vi "NN_Get_Incorrect_Classified_Imgs(RGB)_3D.vi"(4 "# of columns":i32=16, 6 "Dataset":T2={"Inputs Ref."=variant(refnum<data-value> refnum), "Outputs Ref."=refnum, "Dataset_Size"=0, "Dims_In"={"C"=0, "H"=0, "W"=0}, "Dims_Out"=0, "Labels"=[], "File Paths"=[]}, 7 "Labels":string[](array[string]), 8 "error in (no error)":errorcluster, 10 "Predictions":sgl[][](array[numeric]), 11 "MisClassed_idx":i32[](array[numeric])) -> (0 "error out":errorcluster, 3 "Images(GrayScale)":T1[][](array[typedef]))   [LabVIEW 2020]
doc: "Helper VI for analysis.\nReturns Images as intensity graphs with the ground truth and corresponding predictions."
uses:
  <vilib>/Ngene/Deep Learning Toolkit/Toolkit/NN_Data/API/DataSet/DataSet_Types/NN_DataSet(In3D_Out1D).ctl
  <vilib>/Ngene/Deep Learning Toolkit/Toolkit/NN_Data/Controls/DataRef_Types/2D/NN_Data_ref(2D_SGL).ctl
  <vilib>/Ngene/Deep Learning Toolkit/Toolkit/NN_Data/API/NN_Dims(C,H,W).ctl
  Controls/Img_RGB.ctl
  <vilib>/Ngene/Deep Learning Toolkit/Toolkit/NN_Data/subVIs/Dataset/NN_Variant_to_DVR/4D/NN_Data_Variant_to_DVR(4D_SGL).vi
  <vilib>/picture/picture.llb/Draw True-Color Pixmap.vi
  <vilib>/Ngene/Deep Learning Toolkit/Toolkit/Deep_Learning_Toolkit_by_Ngene.lvlib
  <vilib>/vision/NI_Vision_Development_Module.lvlib
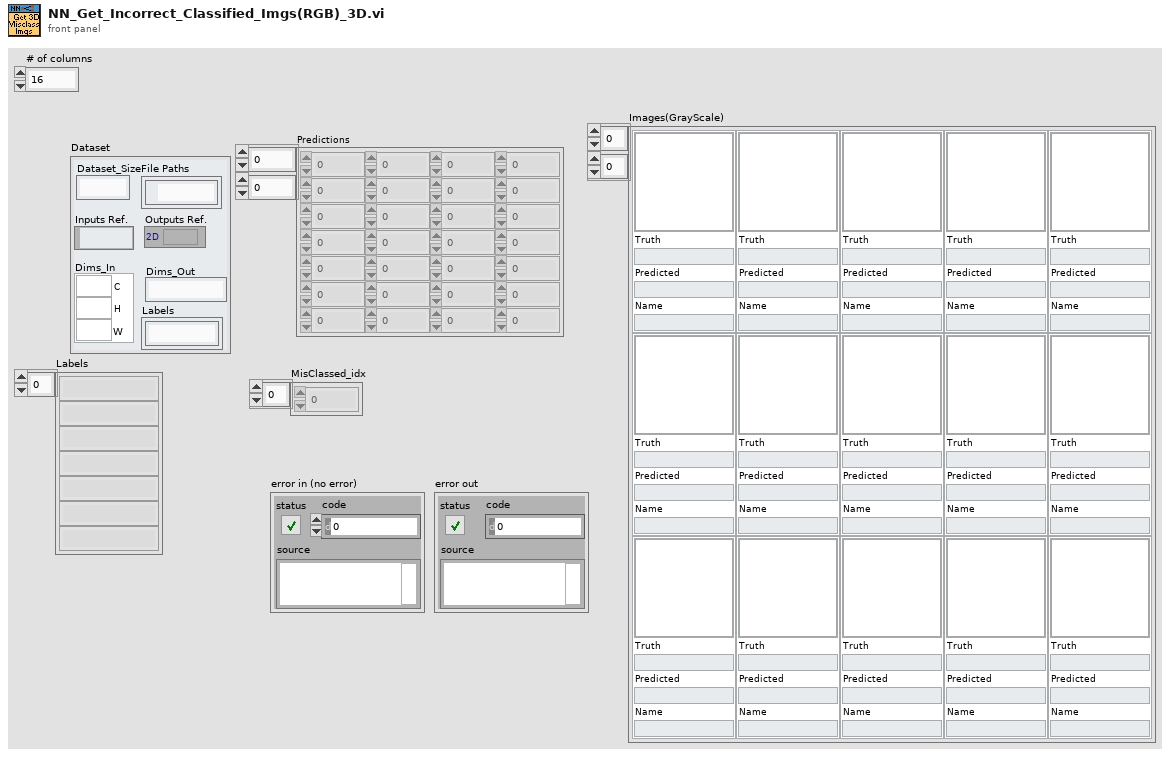
[diagram p1: front panel]
types:
  T1 = typedef "Img_RGB.ctl" = cluster{"image":picture, "Truth":string, "Predicted":string, "Name":string}
  T2 = typedef "Deep_Learning_Toolkit_by_Ngene.lvlib/NN_DataSet(In3D_Out1D).ctl" = cluster{"Inputs Ref.":variant, "Outputs Ref.":T3, "Dataset_Size":i32, "Dims_In":T4, "Dims_Out":i32, "Labels":string[], "File Paths":path[]}
  T3 = typedef "Deep_Learning_Toolkit_by_Ngene.lvlib/NN_Data_ref(2D_SGL).ctl" = refnum<data-value>
  T4 = typedef "Deep_Learning_Toolkit_by_Ngene.lvlib/NN_Dims(C,H,W).ctl" = cluster{"C":i32, "H":i32, "W":i32}
  T5 = typedef "Image Type" = u32
  T6 = typedef "Deep_Learning_Toolkit_by_Ngene.lvlib/NN_Data_ref(4D_SGL).ctl" = refnum<data-value>
  T7 = typedef "IMAQ Image.ctl" = refnum<image>
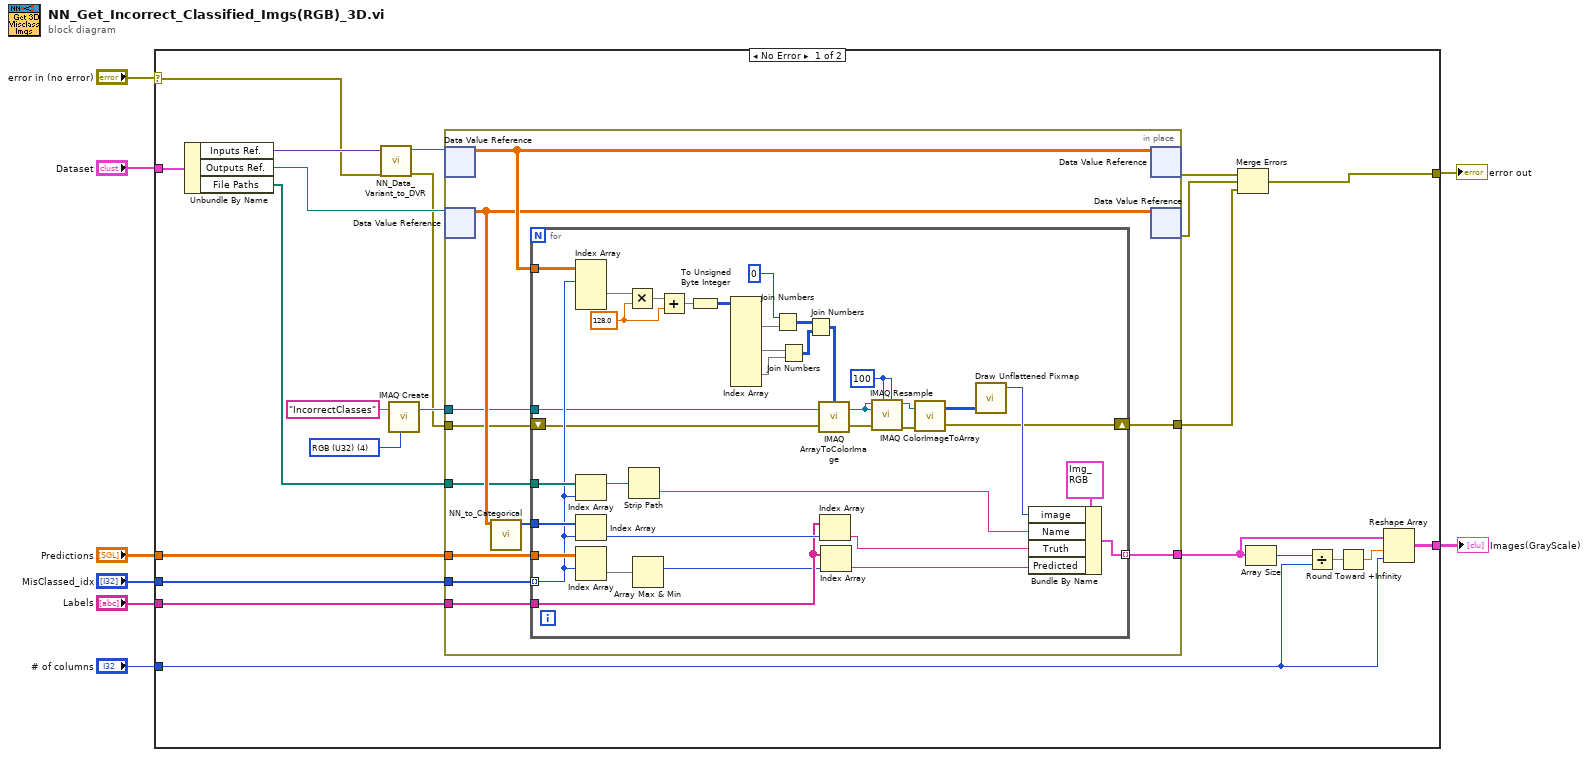
[diagram p0: block diagram]
diagram:
  n1 = case shown="No Error" "error in (no error)" {
    selector: "error in (no error)" -> [w20 w80]
    tunnel: [w31 w80] -> w8
    tunnel: "Dataset" -> [w26 _]
    tunnel: "Predictions" -> [w25 _]
    tunnel: "MisClassed_idx" -> [w24 _]
    tunnel: [w23 _] -> w3
    tunnel: "Labels" -> [w17 _]
    tunnel: "# of columns" -> [w15 _]
    frame No Error {
      w14 = T5 4 items=["Grayscale (U8)", "Grayscale (I16)", "Grayscale (SGL)", "Complex (CSG)", "RGB (U32)", "HSL (U32)", "RGB (U64)", "Grayscale (U16)"] ("Image Type")
      n2 = Unbundle By Name(w26) -> ("Inputs Ref."=w21:variant, "Outputs Ref."=w22:T3, "File Paths"=w16:path[])
      n3 = call-poly <vilib>:"NN_Data_Variant_to_DVR.vi"("error in (no error)"=w20, "Inputs Ref."=w21) -> ("error out"=w11:errorcluster, "DVR(4D_SGL)"=w19:T6)  [unwired: 8 in]
      n4 = call "IMAQ Create"("Image Name"="IncorrectClasses", "Image Type"=w14) -> ("New Image"=w12:T7)  [unwired: 3 in, 1 out]
      n5 = in-place {
        in-place-border: w24 -> [w42]
        in-place-border: w25 -> [w38]
        in-place-border: [w40] -> w27
        in-place-border: w17 -> [w36]
        in-place-border: w16 -> [w35]
        in-place-border: w12 -> [w34]
        in-place-border: w11 -> [w33]
        in-place-border: [w32] -> w10
        n6 = in-place-dvr #1(w19) -> (w41:sgl[][][][])  [unwired: 1 out]
        n7 = in-place-dvr #2(w22) -> (w37:sgl[][])  [unwired: 1 out]
        n8 = call <vilib>:"NN_to_Categorical.vi"("Prediction"=w37) -> ("Label_Idx"=w39:i32[])  [unwired: 10 in]
        n9 = for {
          tunnel: w41 -> [w79]
          tunnel: w42 -> [w56] mode=indexing
          tunnel: w39 -> [w78]
          tunnel: w38 -> [w77]
          tunnel: [w74] -> w40 mode=indexing
          tunnel: w36 -> [w71]
          tunnel: w35 -> [w57]
          tunnel: w34 -> [w52]
          shift-right: [w43] -> w32
          shift-left: w33 -> [w44]
          w49 = 100 ("Y Resolution")
          w66 = sgl 128.0 ("y")
          n10 = Index Array(array=w79, index (dim 0)=w56) -> (element=w68:sgl[][][])  [unwired: 3 in]
          n11 = Index Array(array=w57, index=w56) -> (element=w55:path)
          n12 = Index Array(array=w78, index=w56) -> (element=w73:i32)
          n13 = Index Array(array=w77, index (row)=w56) -> (element=w75:sgl[])  [unwired: 1 in]
          n14 = Multiply(x=w68, y=w66) -> (x*y=w67:sgl[][][])
          n15 = Strip Path(path=w55) -> (name=w54:string)  [unwired: 1 out]
          n16 = Array Max & Min(array=w75) -> (max index (indices)=w70:i32)  [unwired: 3 out]
          n17 = Add(x=w67, y=w66) -> (x+y=w65:sgl[][][])
          n18 = To Unsigned Byte Integer(number=w65) -> (unsigned 8bit integer=w64:u8[][][])
          n19 = Index Array(array=w64) -> (element #1=w63:u8[][], element #2=w61:u8[][], element #3=w60:u8[][])  [unwired: 9 in]
          n20 = Join Numbers(hi=u8 0, lo=w63) -> ((hi.lo)=w59:u16[][])
          n21 = Join Numbers(hi=w61, lo=w60) -> ((hi.lo)=w58:u16[][])
          n22 = Join Numbers(hi=w59, lo=w58) -> ((hi.lo)=w51:u32[][])
          n23 = call "IMAQ ArrayToColorImage"("Image Pixels (U32)"=w51, "Image"=w52, "error in (no error)"=w44) -> ("Image Out"=w47:T7, "error out"=w50:errorcluster)  [unwired: 2 in]
          n24 = Index Array(array=w71, index=w73) -> (element=w72:string)
          n25 = Index Array(array=w71, index=w70) -> (element=w69:string)
          n26 = call "IMAQ Resample"("X Resolution"=w49, "Y Resolution"=w49, "error in (no error)"=w50, "Image Dst"=w47, "Image Src"=w47) -> ("error out"=w46:errorcluster, "Image Dst Out"=w48:T7)  [unwired: 5 in]
          n27 = call "IMAQ ColorImageToArray"("Image"=w48, "error in (no error)"=w46) -> ("Image Pixels (U32)"=w45:u32[][], "error out"=w43:errorcluster)  [unwired: 2 in, 1 out]
          n28 = call-poly <vilib>:"Draw Unflattened Pixmap.vi"("data (RGB format)"=w45) -> ("new picture"=w53:picture)  [unwired: 8 in]
          n29 = Bundle By Name(cluster=T1 {"image"=bytes[0], "Truth"="", "Predicted"="", "Name"=""}, "image"=w53, "Name"=w54, "Truth"=w72, "Predicted"=w69) -> (w74:T1)
        }
        n30 = in-place-dvr #1(w41) -> (w18:errorcluster)  [unwired: 1 out]
        n31 = in-place-dvr #2(w37) -> (w9:errorcluster)  [unwired: 1 out]
      }
      n32 = Merge Errors(w18, w9, w10) -> (w31:errorcluster)
      n33 = Array Size(array=w27) -> (size(s)=w30:i32)
      n34 = Divide(x=w30, y=w15) -> (x/y=w29:dbl)
      n35 = Round Toward +Infinity(x=w29) -> (ceil(x): smallest int >= x=w28:dbl)
      n36 = Reshape Array(w27, w28, w15) -> (w23:T1[][])
    }
    frame Error {
    }
  }
  "error out" <- w8
  "Images(GrayScale)" <- w3
